vi "mux.rem.vi"(11 "# of existing\nitems 3":u8) -> (3 "y":i8)   [LabVIEW 2020]
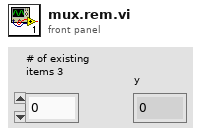
[diagram p1: front panel]
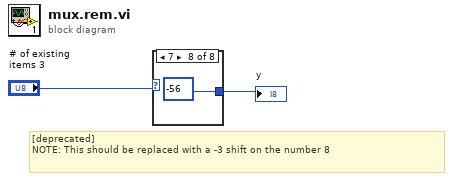
[diagram p0: block diagram]
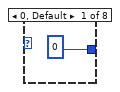
[diagram p2: hidden frame]
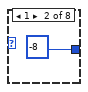
[diagram p3: hidden frame]
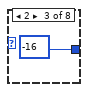
[diagram p4: hidden frame]
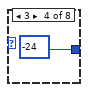
[diagram p5: hidden frame]
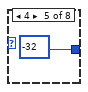
[diagram p6: hidden frame]
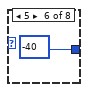
[diagram p7: hidden frame]
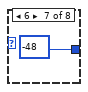
[diagram p8: hidden frame]
diagram:
  # "[deprecated]\nNOTE: This should be replaced with a -3 shift on the number 8"
  n1 = case shown="7" "# of existing\nitems 3" {
    tunnel: [i8 0 ("y") i8 -8 ("y") i8 -16 ("y") i8 -24 ("y") i8 -32 ("y") i8 -40 ("y") i8 -48 ("y") i8 -56 ("y")] -> w2
    frame 0, Default {
    }
    frame 1 {
    }
    frame 2 {
    }
    frame 3 {
    }
    frame 4 {
    }
    frame 5 {
    }
    frame 6 {
    }
    frame 7 {
    }
  }
  "y" <- w2
